vi "Twist-Handle Values.vi"() -> (0 "Twist-Handle":T1)   [LabVIEW 2014]
uses:
  <vilib>/Rock Robotics/Network Tables/SD Write Boolean Array.vi
  <vilib>/Rock Robotics/Network Tables/SD Write Numeric Array.vi
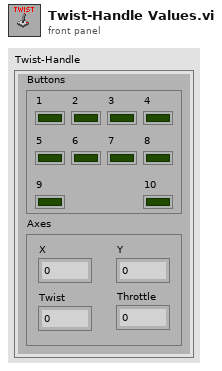
[diagram p1: front panel]
types:
  T1 = cluster{"Buttons":cluster{"1":bool, "2":bool, "3":bool, "4":bool, "5":bool, "6":bool, "7":bool, "8":bool, "9":bool, "10":bool}, "Axes":cluster{"X":dbl, "Y":dbl, "Twist":dbl, "Throttle":dbl}}
  T2 = cluster{"Boolean":bool, "Boolean":bool, "Boolean":bool, "Boolean":bool, "Boolean":bool, "Boolean":bool, "Boolean":bool, "Boolean":bool, "Boolean":bool, "Boolean":bool}
  T3 = cluster{"Numeric":dbl, "Numeric":dbl, "Numeric":dbl, "Numeric":dbl}
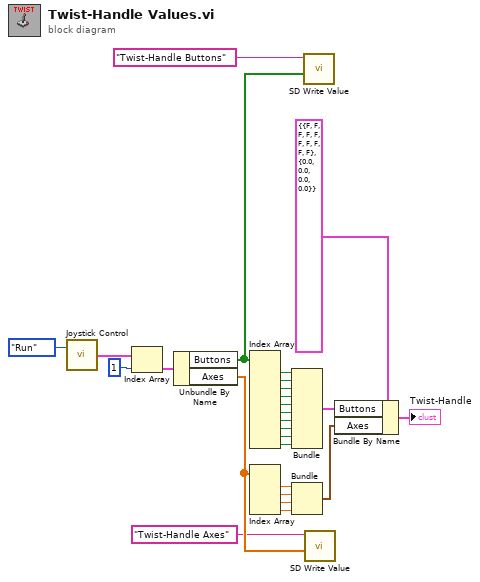
[diagram p0: block diagram]
diagram:
  n1 = call "Joystick Control.vi"("Mode"=enum8{"Start", "Run", "Finish"}."Run") -> ("Joysticks"=w25:cluster{"Buttons":bool[], "Axes":dbl[]}[])  [unwired: 1 in]
  n2 = Index Array(array=w25, index=1) -> (element=w24:cluster{"Buttons":bool[], "Axes":dbl[]})
  n3 = Unbundle By Name(w24) -> ("Buttons"=w4:bool[], "Axes"=w2:dbl[])
  n4 = Index Array(array=w4) -> (element #1=w22:bool, element #2=w23:bool, element #3=w14:bool, element #4=w15:bool, element #5=w16:bool, element #6=w17:bool, element #7=w18:bool, element #8=w19:bool, element #9=w20:bool, element #10=w21:bool)  [unwired: 10 in]
  n5 = Index Array(array=w2) -> (element #1=w12:dbl, element #2=w13:dbl, element #3=w10:dbl, element #4=w11:dbl)  [unwired: 4 in]
  n6 = Bundle("Boolean"=w22, "Boolean"=w23, "Boolean"=w14, "Boolean"=w15, "Boolean"=w16, "Boolean"=w17, "Boolean"=w18, "Boolean"=w19, "Boolean"=w20, "Boolean"=w21) -> (w9:T2)  [unwired: 1 in]
  n7 = Bundle("Numeric"=w12, "Numeric"=w13, "Numeric"=w10, "Numeric"=w11) -> (w8:T3)  [unwired: 1 in]
  n8 = call-poly <vilib>:"SD Write Value.vi"("Boolean Array"=w4, "Name"="Twist-Handle Buttons") -> ()  [unwired: 8 in, 2 out]
  n9 = call-poly <vilib>:"SD Write Value.vi"("Numeric Array"=w2, "Name"="Twist-Handle Axes") -> ()  [unwired: 8 in, 2 out]
  n10 = Bundle By Name(cluster=T1 {"Buttons"={"1"=FALSE, "2"=FALSE, "3"=FALSE, "4"=FALSE, "5"=FALSE, "6"=FALSE, "7"=FALSE, "8"=FALSE, "9"=FALSE, "10"=FALSE}, "Axes"={"X"=0.0, "Y"=0.0, "Twist"=0.0, "Throttle"=0.0}} ("Twist-Handle"), "Buttons"=w9, "Axes"=w8) -> (→"Twist-Handle":T1)
